vi "Configure IF Gain (Swept SA).vi"(8 "error in (no error)":errorcluster, 9 "FFT IF Gain (0: Auto)":i32(ring) items=["Auto", "Autorange", "Low Gain", "High Gain"], 10 "Swept IF Gain (0: Auto)":i32(ring) items=["Auto", "Low Gain", "High Gain"], 11 "VISA resource name":refnum<visa-resource-name>) -> (0 "error out":errorcluster, 3 "VISA resource name out":refnum<visa-resource-name>)   [LabVIEW 2018, in "Agilent MXA Series.lvlib"]
doc: "Configures the IF gain in Swept SA measurement type."
uses:
  Agilent MXA Series.lvlib
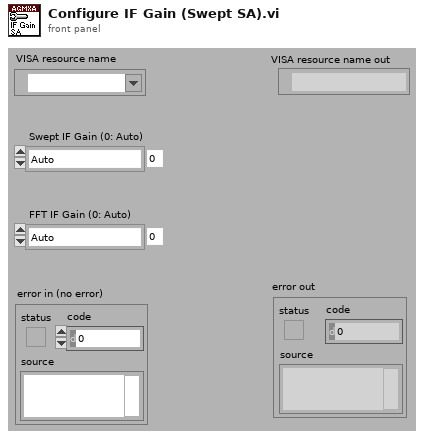
[diagram p1: front panel]
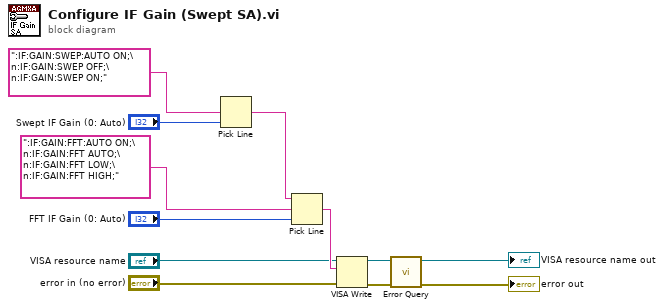
[diagram p0: block diagram]
diagram:
  n1 = Pick Line(multi-line string=":IF:GAIN:SWEP:AUTO ON;\n:IF:GAIN:SWEP OFF;\n:IF:GAIN:SWEP ON;", line index="Swept IF Gain (0: Auto)") -> (output string=w8:string)  [unwired: 1 in]
  n2 = Pick Line(string ("")=w8, multi-line string=":IF:GAIN:FFT:AUTO ON;\n:IF:GAIN:FFT AUTO;\n:IF:GAIN:FFT LOW;\n:IF:GAIN:FFT HIGH;", line index="FFT IF Gain (0: Auto)") -> (output string=w7:string)
  n3 = VISA Write(VISA resource name="VISA resource name", write buffer=w7, error in (no error)="error in (no error)") -> (VISA resource name out=w4:refnum<visa-resource-name>, error out=w5:errorcluster)  [unwired: 1 out]
  n4 = call "Error Query.vi"("error in (no error)"=w5, "VISA resource name"=w4) -> ("error out"=→"error out":errorcluster, "VISA resource name out"=→"VISA resource name out":refnum<visa-resource-name>)  [unwired: 6 in, 2 out]
